vi "serialrecv.vi"() -> ()   [LabVIEW 2012]
uses:
  <vilib>/Instr/_visa.llb/VISA Configure Serial Port (Instr).vi
panel:
  out "Waveform Graph":dbl[](graph)
  out "data":dbl[][](array[numeric]) format="%#_17g"
  out "value":cluster{"time":i32, "alt":sgl}
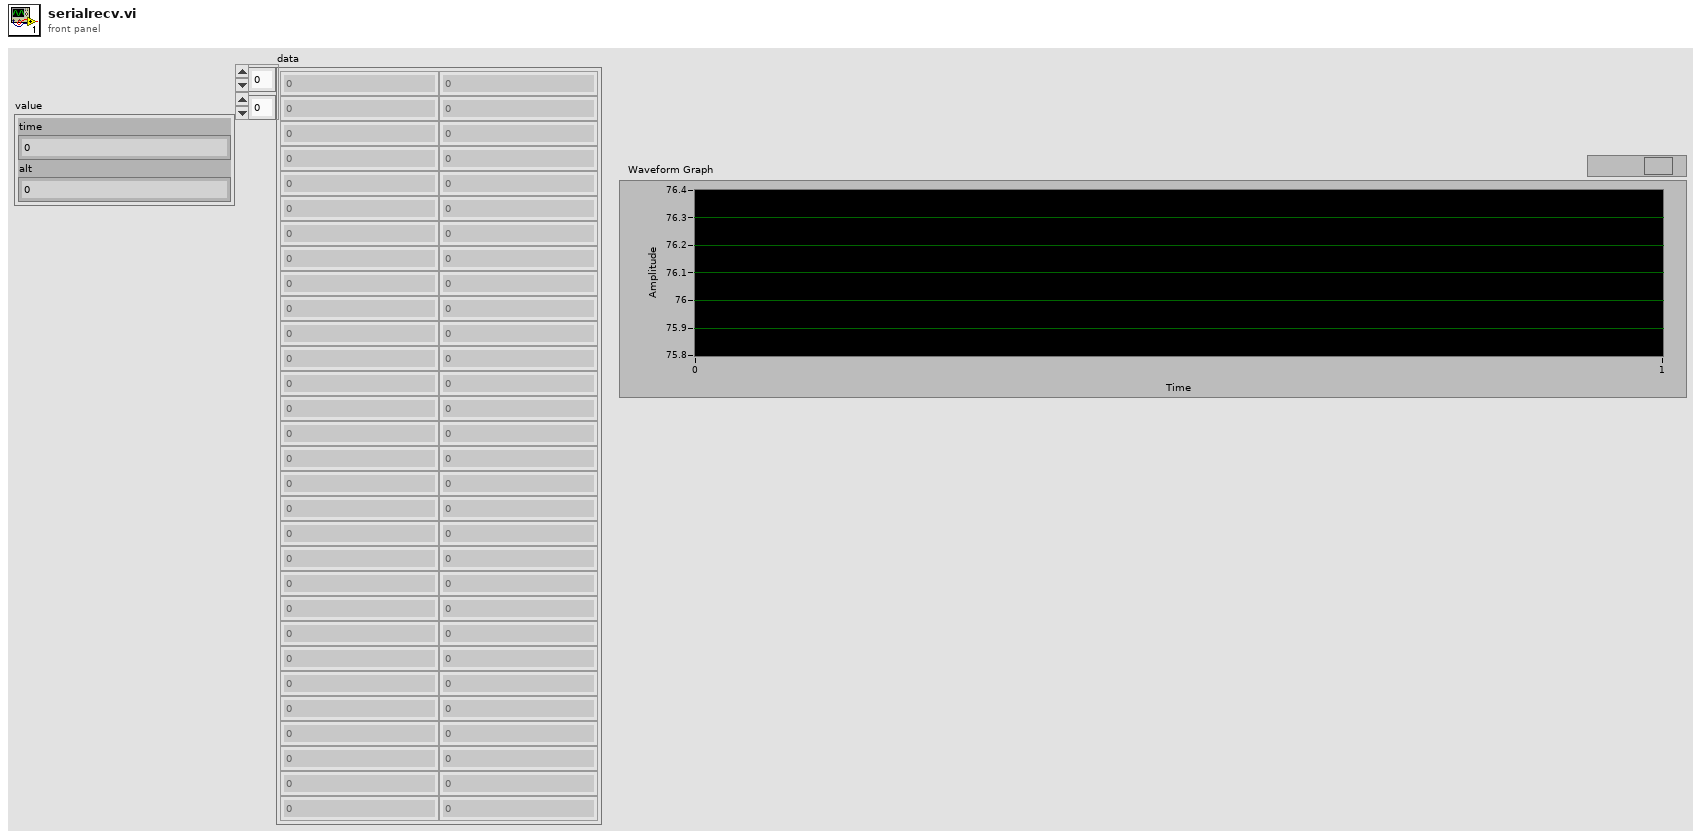
[diagram p1: front panel]
types:
  T1 = enum16{"big-endian, network order", "native, host order", "little-endian"}
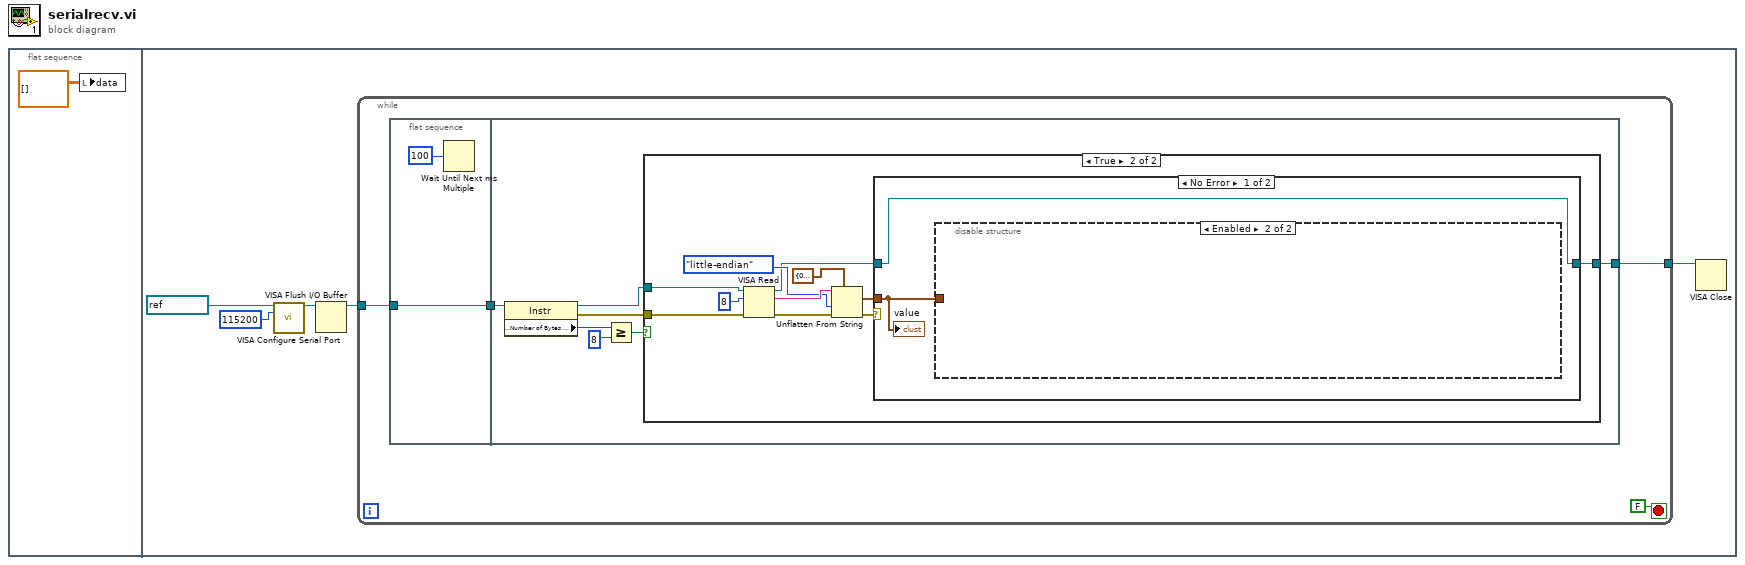
[diagram p0: block diagram]
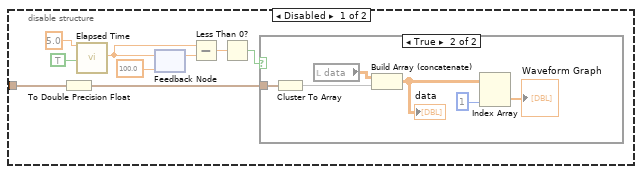
[diagram p3: hidden frame]
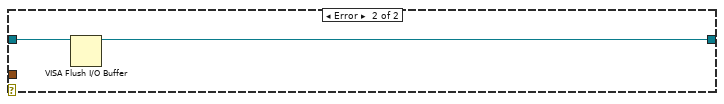
[diagram p5: hidden frame]
diagram:
  n1 = flat-sequence {
    frame #0 {
      n2 = local write "data"(dbl[][] [] ("data")) -> ()
    }
    frame #1 {
      n3 = call-poly "VISA Configure Serial Port"("VISA resource name"=refnum<visa-resource-name> "COM7", "baud rate (9600)"=u32 115200) -> ("VISA resource name out"=w3:refnum<visa-resource-name>)  [unwired: 7 in, 6 out]
      n4 = VISA Flush I/O Buffer(VISA resource name=w3) -> (VISA resource name out=w2:refnum<visa-resource-name>)  [unwired: 2 in, 1 out]
      n5 = while {
        tunnel: w2 -> [w8]
        tunnel: [w9] -> w4
        stop <- FALSE ("Boolean") stop-if-true
        n6 = flat-sequence {
          tunnel: w8 -> [w12]
          tunnel: [w12] -> w7
          tunnel: [w19] -> w9
          tunnel: w7 -> [w18]
          frame #0 {
            n7 = Wait Until Next ms Multiple(millisecond multiple=u32 100) -> ()  [unwired: 1 out]
          }
          frame #1 {
            n8 = property class="Instr"(reference=w18) -> (reference out=w17:refnum<visa-resource-name>, error out=w13:errorcluster, "Serial Settings:Number of Bytes at Serial Port"=w16:u32)  [unwired: 1 in]
            n9 = Greater Or Equal?(x=w16, y=u32 8) -> (x >= y?=w14:bool)
            n10 = case shown="True" w14 {
              tunnel: [w20 w25] -> w19
              tunnel: w17 -> [w20 w27]
              tunnel: w13 -> [_ w22]
              frame False {
              }
              frame True {
                n11 = VISA Read(VISA resource name=w27, byte count=u32 8, error in (no error)=w22) -> (VISA resource name out=w24:refnum<visa-resource-name>, read buffer=w29:string, error out=w23:errorcluster)  [unwired: 1 out]
                n12 = Unflatten From String(type=cluster{"time":i32, "alt":sgl} {"time"=0, "alt"=0.0}, binary string=w29, byte order (0:big-endian, network order)=T1."little-endian", error in (no error)=w23) -> (value=w21:cluster{"time":i32, "alt":sgl}, error out=w26:errorcluster)  [unwired: 1 in, 1 out]
                n13 = case shown="No Error" w26 {
                  tunnel: [w33 w49] -> w25
                  tunnel: w24 -> [w33 w50]
                  tunnel: w21 -> [w32 _]
                  frame No Error {
                    n14 = disable-structure shown="Enabled" {
                      disable-tunnel: w32 -> [w42 _]
                      frame Disabled {
                        n15 = To Double Precision Float(number=w42) -> (double precision float=w41:cluster{"time":dbl, "alt":dbl})
                        n16 = call "Elapsed Time"("Time Target (s)"=5.0, "Auto Reset"=TRUE) -> ("Elapsed Time (s)"=w37:dbl)  [unwired: 10 in, 7 out]
                        n17 = feedback #1(100.0 ("Elapsed Time (s)")) -> (w38:dbl)
                        n18 = feedback-in #1(w37) -> ()
                        n19 = Subtract(x=w37, y=w38) -> (x-y=w36:dbl)
                        n20 = Less Than 0?(x=w36) -> (x < 0?=w35:bool)
                        n21 = case shown="True" w35 {
                          tunnel: w41 -> [_ w48]
                          frame False {
                          }
                          frame True {
                            n22 = Cluster To Array(cluster=w48) -> (array=w47:dbl[])
                            n23 = local read "data"() -> (w46:dbl[][])
                            n24 = Build Array (concatenate)(w46, w47) -> (w45:dbl[][])
                            "data" <- w45
                            n25 = Index Array(array=w45, index (col)=1 ("disabled index (col)")) -> (element=→"Waveform Graph":dbl[])  [unwired: 1 in]
                          }
                        }
                      }
                      frame Enabled {
                      }
                    }
                    "value" <- w32
                  }
                  frame Error {
                    n26 = VISA Flush I/O Buffer(VISA resource name=w50) -> (VISA resource name out=w49:refnum<visa-resource-name>)  [unwired: 2 in, 1 out]
                  }
                }
              }
            }
          }
        }
      }
      n27 = VISA Close(VISA resource name=w4) -> ()  [unwired: 1 in, 1 out]
    }
  }
